vi "Destructor.vi"(8 "error in":errorcluster, 11 "Owlstone OVG-4 in":refnum<class "Owlstone GEN-SYS.lvclass">) -> (0 "error out":errorcluster, 3 "Owlstone OVG-4 out":refnum<class "Owlstone GEN-SYS.lvclass">)   [LabVIEW 2011, in "Owlstone GEN-SYS.lvclass"]
uses:
  Owlstone GEN-SYS.lvclass
  Owlstone GEN-SYS.lvclass/Owlstone GEN-SYS.ctl
  Eurotherm 3200 PID Controller/Eurotherm 3200 PID Controller.lvclass
  Michell Easidew/Michell Easidew.lvclass
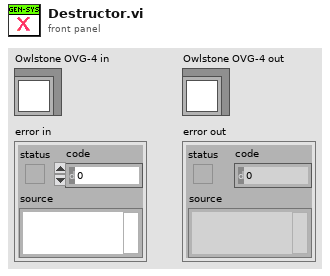
[diagram p1: front panel]
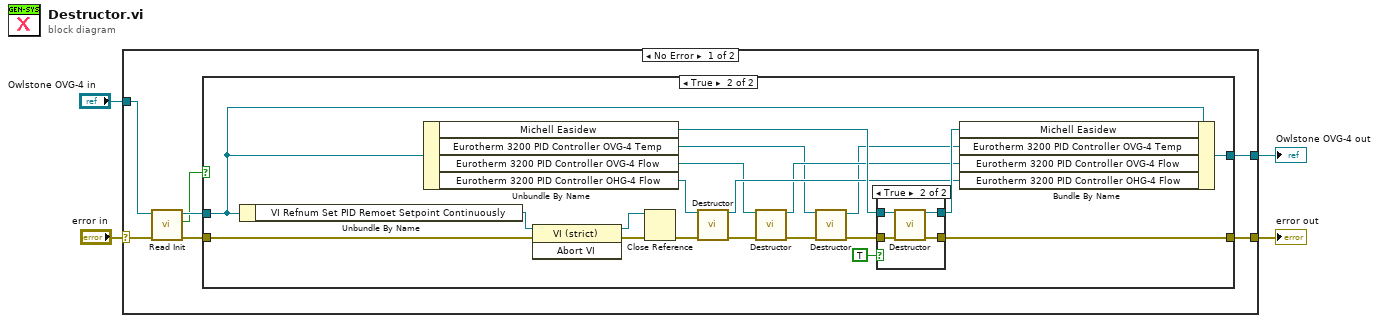
[diagram p0: block diagram]
diagram:
  n1 = case shown="No Error" "error in" {
    selector: "error in" -> [w9 w41]
    tunnel: [w11 w41] -> w3
    tunnel: [w10 w40] -> w1
    tunnel: "Owlstone OVG-4 in" -> [w7 w40]
    frame No Error {
      n2 = call-dynamic "Read Init.vi"("error in (no error)"=w9, "Vapour Generator in"=w7) -> ("error out"=w8:errorcluster, "Init"=w5:bool, "Vapour Generator out"=w6:refnum<class "Owlstone GEN-SYS.lvclass">)  [unwired: 7 in]
      n3 = case shown="True" w5 {
        tunnel: [w12 w32] -> w11
        tunnel: [w13 w30] -> w10
        tunnel: w8 -> [w12 w19]
        tunnel: w6 -> [w13 w18]
        frame False {
        }
        frame True {
          n4 = Unbundle By Name(w18) -> ("VI Refnum Set PID Remoet Setpoint Continuously"=w20:refnum<vi>)
          n5 = Unbundle By Name(w18) -> ("Michell Easidew"=w33:refnum<class "Michell Easidew.lvclass">, "Eurotherm 3200 PID Controller OVG-4 Temp"=w24:refnum<class "Eurotherm 3200 PID Controller.lvclass">, "Eurotherm 3200 PID Controller OVG-4 Flow"=w26:refnum<class "Eurotherm 3200 PID Controller.lvclass">, "Eurotherm 3200 PID Controller OHG-4 Flow"=w29:refnum<class "Eurotherm 3200 PID Controller.lvclass">)
          n6 = invoke class="VI (strict)" method="Abort VI"(reference=w20, error in=w19) -> (reference out=w16:refnum<vi>, error out=w17:errorcluster)  [unwired: 1 in, 1 out]
          n7 = Close Reference(reference=w16, error in (no error)=w17) -> (error out=w15:errorcluster)
          n8 = call-dynamic "Destructor.vi"("error in (no error)"=w15, "Eurotherm 3200 PID Controller in"=w29) -> ("error out"=w27:errorcluster, "Eurotherm 3200 PID Controller out"=w28:refnum<class "Eurotherm 3200 PID Controller.lvclass">)  [unwired: 8 in]
          n9 = call-dynamic "Destructor.vi"("error in (no error)"=w27, "Eurotherm 3200 PID Controller in"=w26) -> ("error out"=w22:errorcluster, "Eurotherm 3200 PID Controller out"=w25:refnum<class "Eurotherm 3200 PID Controller.lvclass">)  [unwired: 8 in]
          n10 = call-dynamic "Destructor.vi"("error in (no error)"=w22, "Eurotherm 3200 PID Controller in"=w24) -> ("error out"=w21:errorcluster, "Eurotherm 3200 PID Controller out"=w23:refnum<class "Eurotherm 3200 PID Controller.lvclass">)  [unwired: 8 in]
          n11 = case shown="True" TRUE {
            tunnel: w33 -> [w35 w39]
            tunnel: [w34 w38] -> w32
            tunnel: [w35 w37] -> w31
            tunnel: w21 -> [w34 w36]
            frame False {
            }
            frame True {
              n12 = call-dynamic "Destructor.vi"("error in"=w36, "Michell Easydew in"=w39) -> ("error out"=w38:errorcluster, "Michell Easydew out"=w37:refnum<class "Michell Easidew.lvclass">)  [unwired: 8 in]
            }
          }
          n13 = Bundle By Name(cluster=w18, "Michell Easidew"=w31, "Eurotherm 3200 PID Controller OVG-4 Temp"=w23, "Eurotherm 3200 PID Controller OVG-4 Flow"=w25, "Eurotherm 3200 PID Controller OHG-4 Flow"=w28) -> (w30:refnum<class "Owlstone GEN-SYS.lvclass">)
        }
      }
    }
    frame Error {
    }
  }
  "error out" <- w3
  "Owlstone OVG-4 out" <- w1
